vi "IniTriggerTime.vi"(8 "error in":errorcluster, 10 "Report_Time section":string="Modbus", 11 "INI file path":path=path "C:/Users/User/Desktop/YDX701_TDC/iniData/TDC_IniData.ini") -> (0 "error out":errorcluster, 1 "搬移延遲":i32, 2 "延遲(分)":i32, 3 "時間(點, 區間)":i32[][](array[numeric]))   [LabVIEW 2019]
uses:
  33fdea91-c140-4aad-a887-90c630a000af.vi
  <vilib>/Array/Sort 2D Array - Pop Stack.vi
  <vilib>/Array/Sort 2D Array - Push Stack.vi
  33fdea91-c140-4aad-a887-90c630a000af.vi/17345d16-769b-40a7-8fcc-cf5bb879e1e6.vi
  33fdea91-c140-4aad-a887-90c630a000af.vi/15f03ce1-14e8-4f79-a87e-8e5a0c5e3a0c.vi
  <vilib>/Utility/config.llb/Read Key (String).vi
  <vilib>/Utility/config.llb/Read Key (I32).vi
  <vilib>/Utility/config.llb/NI_LVConfig.lvlib
panel:
  out "array":string[](array[string])
  out "(時間點,區間)":string
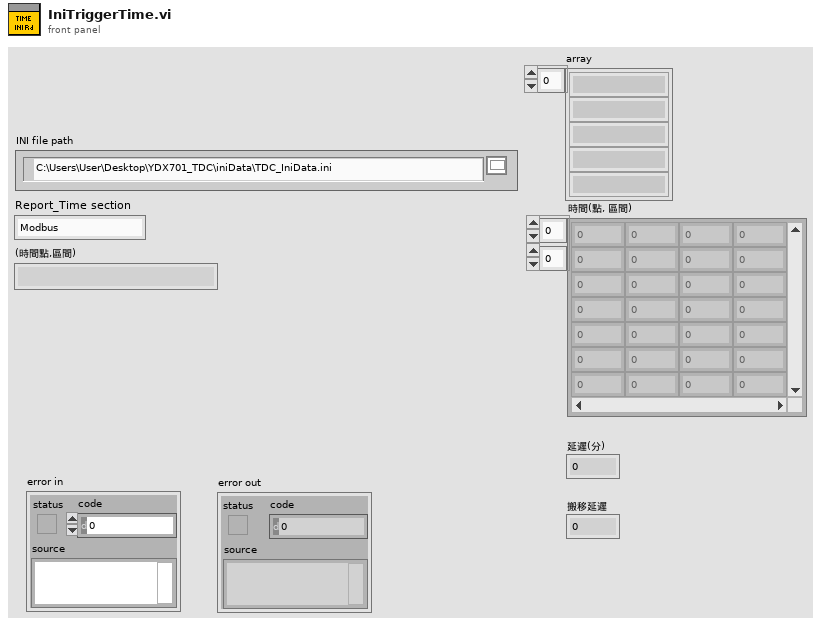
[diagram p1: front panel]
types:
  T1 = typedef "NI_LVConfig.lvlib/Config Data RefNum.ctl" = refnum<k1>
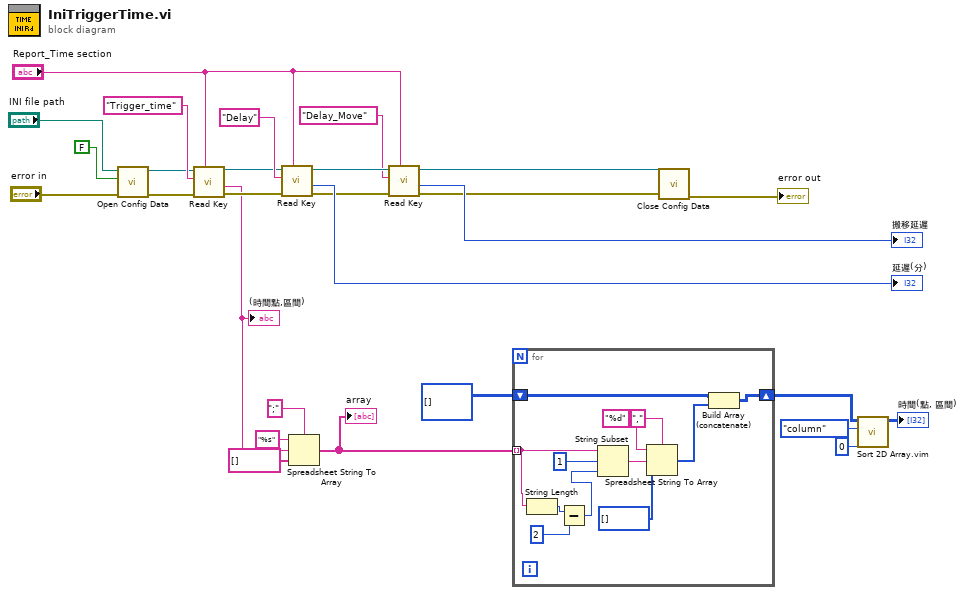
[diagram p0: block diagram]
diagram:
  n1 = call <vilib>:"Open Config Data.vi"("error in (no error)"="error in", "create file if necessary (T)"=FALSE ("create file if necessary? (T)"), "configuration file path"="INI file path") -> ("error out"=w26:errorcluster, "refnum"=w24:T1)  [unwired: 6 in, 1 out]
  n2 = call-poly <vilib>:"Read Key.vi"("section"="Report_Time section", "error in (no error)"=w26, "key"="Trigger_time", "refnum"=w24) -> ("error out"=w19:errorcluster, "value"=w14:string, "refnum out"=w20:T1)  [unwired: 2 in, 3 out]
  "(時間點,區間)" <- w14
  n3 = call-poly <vilib>:"Read Key.vi"("section"="Report_Time section", "error in (no error)"=w19, "key"="Delay", "refnum"=w20) -> ("error out"=w6:errorcluster, "value"=→"延遲(分)":i32, "refnum out"=w7:T1)  [unwired: 1 in, 4 out]
  n4 = Spreadsheet String To Array(delimiter (Tab)=";", format string="%s", spreadsheet string=w14, array type (2D Dbl)=string[] []) -> (array=w13:string[])
  "array" <- w13
  n5 = call-poly <vilib>:"Read Key.vi"("section"="Report_Time section", "error in (no error)"=w6, "key"="Delay_Move", "refnum"=w7) -> ("error out"=w1:errorcluster, "value"=→"搬移延遲":i32, "refnum out"=w2:T1)  [unwired: 1 in, 4 out]
  n6 = for {
    tunnel: w13 -> [w39] mode=indexing
    shift-right: [w29] -> w11
    shift-left: i32[][] [] ("array type (2D Dbl)") -> [w31]
    n7 = String Length(string=w39) -> (length=w38:i32)
    n8 = Subtract(x=w38, y=2) -> (x-y=w36:i32)
    n9 = String Subset(string=w39, offset (0)=1, length (rest)=w36) -> (substring=w35:string)
    n10 = Spreadsheet String To Array(delimiter (Tab)=",", format string="%d", spreadsheet string=w35, array type (2D Dbl)=i32[] []) -> (array=w30:i32[])
    n11 = Build Array (concatenate)(w31, w30) -> (w29:i32[][])
  }
  n12 = call <vilib>:"Close Config Data.vi"("error in (no error)"=w1, "refnum"=w2) -> ("error out"=→"error out":errorcluster)  [unwired: 1 in, 8 out]
  n13 = call "Sort 2D Array.vim"("index"=0, "dimension to index (column)"=enum16{"column", "row"}."column", "2D array"=w11) -> ("sorted 2D array"=→"時間(點, 區間)":i32[][])  [unwired: 7 in, 1 out]
